vi "Set API.vi"(8 "error in (no error)":errorcluster, 10 "Actor API":refnum<class "Actor API.lvclass">, 11 "Template Artifex in":refnum<class "Template.lvclass">) -> (0 "error out":errorcluster, 3 "Template Artifex out":refnum<class "Template.lvclass">)   [LabVIEW 2020, in "Artifex Template.lvlib" / "Template.lvclass"]
uses:
  Template.lvclass
  Template API/Template API.lvclass
  Artifex/Actor Proxy/Actor API.lvclass
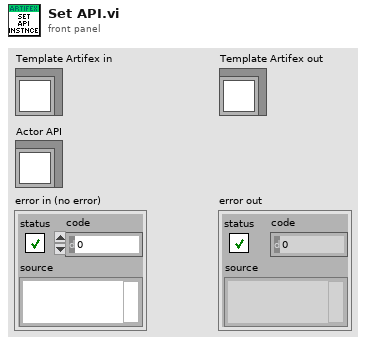
[diagram p1: front panel]
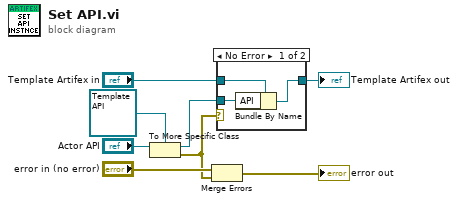
[diagram p0: block diagram]
diagram:
  n1 = To More Specific Class(target class=refnum<class "Template API.lvclass"> refnum ("API"), reference="Actor API") -> (specific class reference=w5:refnum<class "Template API.lvclass">, error out=w1:errorcluster)  [unwired: 1 in]
  n2 = Merge Errors("error in (no error)", w1) -> (→"error out":errorcluster)
  n3 = case shown="No Error" w1 {
    tunnel: w5 -> [w11 _]
    tunnel: "Template Artifex in" -> [w10 w12]
    tunnel: [w9 w12] -> w3
    frame No Error {
      n4 = Bundle By Name(cluster=w10, "API"=w11) -> (w9:refnum<class "Template.lvclass">)
    }
    frame Error {
    }
  }
  "Template Artifex out" <- w3
